vi "Camera Begin.vi"   [LabVIEW 2012]
uses:
  <vilib>/Rock Robotics/SystemInterfaces/DIO/FPGA_DIOPWMChannel.ctl
  <vilib>/Rock Robotics/SystemInterfaces/Typedef/FPGA_TypedefDigitalModule.ctl
  <vilib>/Rock Robotics/WPI/Joystick/WPI_JoystickDeviceEnum.ctl
types:
  T1 = typedef "WPI_JoystickDeviceEnum.ctl" = enum16{"USB 1", "USB 2", "USB 3", "USB 4", "Kinect 1", "Kinect 2"}
  T2 = typedef "FPGA_DIOPWMChannel.ctl" = enum8{"PWM 1", "PWM 2", "PWM 3", "PWM 4", "PWM 5", "PWM 6", "PWM 7", "PWM 8", "PWM 9", "PWM 10", "Invalid"}
  T3 = typedef "FPGA_TypedefDigitalModule.ctl" = enum16{"Digital Module 1", "Digital Module 2"}
  T4 = typedef "WPI_JoystickDevRef.ctl" = cluster{"Device":T1}
  T5 = typedef "WPI_ServoDeviceRef.ctl" = cluster{"DeviceStatus":errorcluster, "Digital Module":T3, "PWM Channel":T2, "DeadBand":T6}
  T6 = typedef "WPI_PWMDeadband.ctl" = cluster{"Name":string, "maxPositivePwm":i32, "minPositivePwm":i32, "centerPwm":i32, "maxNegativePwm":i32, "minNegativePwm":i32, "angularRange":u16}
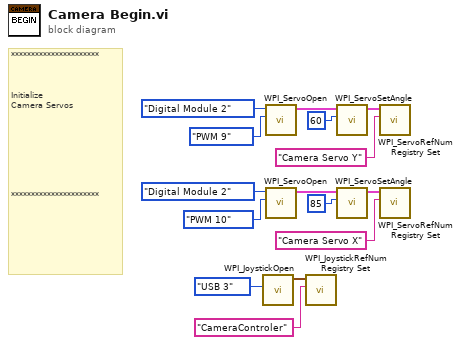
[diagram p0: block diagram]
diagram:
  # "**********************\n\n\n\nInitialize\nCamera Servos\n\n\n\n\n\n\n\n\n**********************"
  n1 = call <vilib>:"WPI_JoystickOpen.vi"("JoystickDevice"=WPI_JoystickDeviceEnum."USB 3") -> ("JoystickDevRef"=w2:T4)  [unwired: 10 in]
  n2 = call <vilib>:"WPI_ServoOpen.vi"("PWM Channel"=FPGA_DIOPWMChannel."PWM 9", "Digital Module (Module 1)"=FPGA_TypedefDigitalModule."Digital Module 2") -> ("ServoDeviceRef"=w13:T5)  [unwired: 8 in, 1 out]
  n3 = call <vilib>:"WPI_ServoOpen.vi"("PWM Channel"=FPGA_DIOPWMChannel."PWM 10", "Digital Module (Module 1)"=FPGA_TypedefDigitalModule."Digital Module 2") -> ("ServoDeviceRef"=w6:T5)  [unwired: 8 in, 1 out]
  n4 = call <vilib>:"WPI_JoystickRefNum Registry Set.vi"("refnum name"="CameraControler", "JoystickDevRef"=w2) -> ()  [unwired: 8 in, 2 out]
  n5 = call <vilib>:"WPI_ServoSetAngle.vi"("Angle"=60, "ServoDeviceRef"=w13) -> ("ServoDeviceRef"=w14:T5)  [unwired: 8 in, 1 out]
  n6 = call <vilib>:"WPI_ServoSetAngle.vi"("Angle"=85, "ServoDeviceRef"=w6) -> ("ServoDeviceRef"=w5:T5)  [unwired: 8 in, 1 out]
  n7 = call <vilib>:"WPI_ServoRefNum Registry Set.vi"("refnum name"="Camera Servo Y", "ServoDeviceRef"=w14) -> ()  [unwired: 8 in, 2 out]
  n8 = call <vilib>:"WPI_ServoRefNum Registry Set.vi"("refnum name"="Camera Servo X", "ServoDeviceRef"=w5) -> ()  [unwired: 8 in, 2 out]
